vi "Human VOG.vi"(0 "3D (unticked 2D) processing":bool, 5 "Bin (unticked Mon) ocular processing":bool, 9 "Interpolate Timebase (Hz)":i32=250, 11 "Gyro scaling":dbl=200.0) -> (15 "Data Output":T1 {"Data Channels" format="%.2f"})   [LabVIEW 2013]
uses:
  <vilib>/Analysis/_algsub.llb/Real PseudoInverse Matrix.vi
  <vilib>/Utility/file.llb/Read From Spreadsheet File (DBL).vi
  comm/fick-matrix/fick-matrix.lvlib
  <vilib>/Analysis/NI_AALPro.lvlib
  comm/quaternion/quaternion.lvlib
panel:
  in  "stop":bool
  # "Human VOG System"
  # "By Americo Migliaccio 17-12-2008"
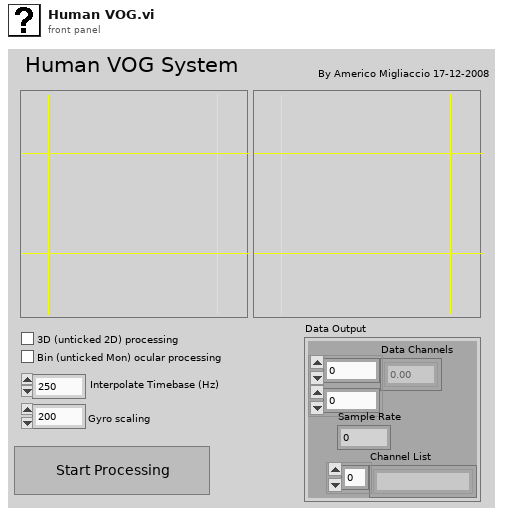
[diagram p1: front panel]
types:
  T1 = cluster{"Data Channels":dbl[][], "Sample Rate":i32, "Channel List":string[]}
  T2 = typedef "NI_Matrix.lvlib/RealMatrix.ctl" = dbl[][]
  T3 = cluster{dbl[][], "Interpolate Timebase (Hz)":i32, string[]}
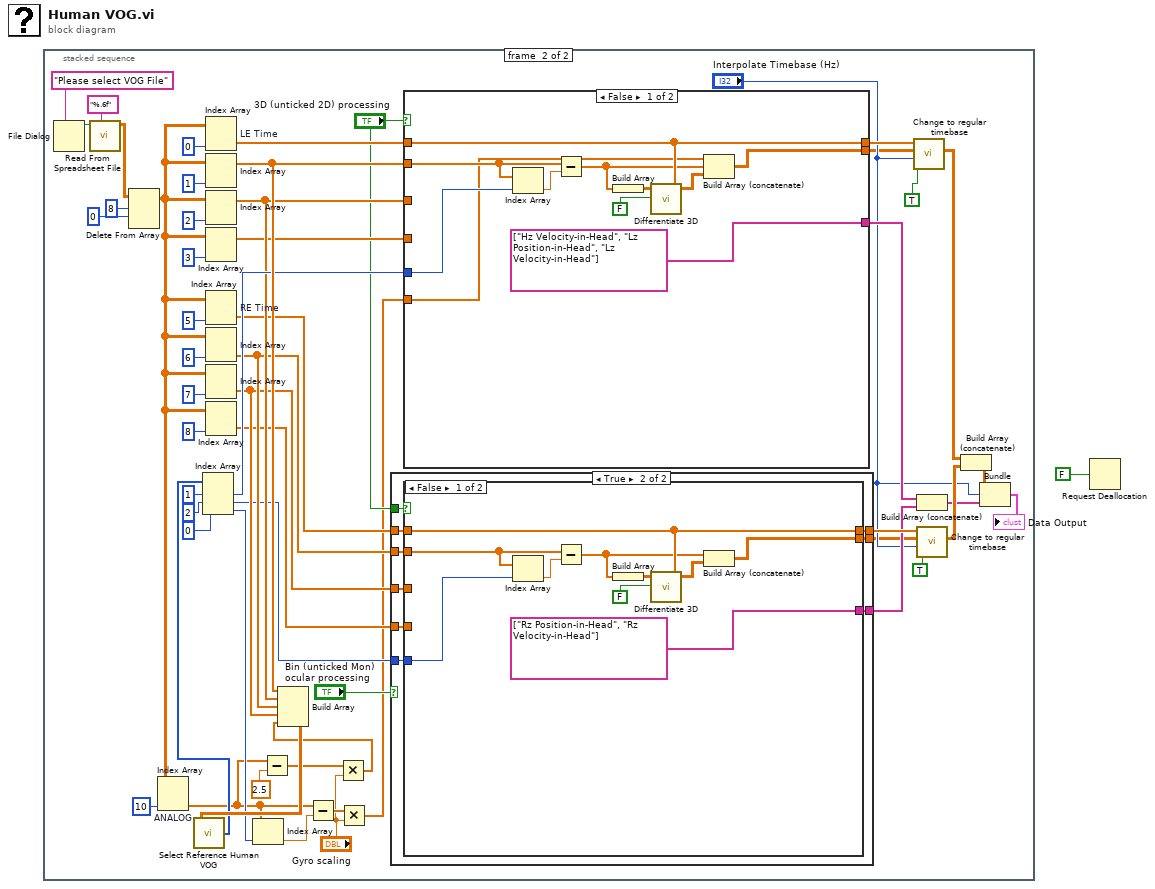
[diagram p0: block diagram]
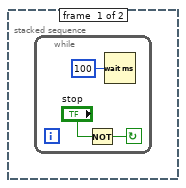
[diagram p2: hidden frame]
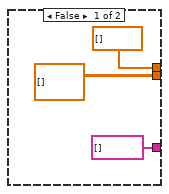
[diagram p3: hidden frame]
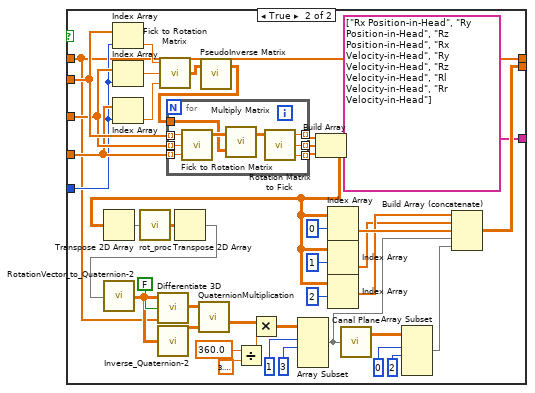
[diagram p4: hidden frame]
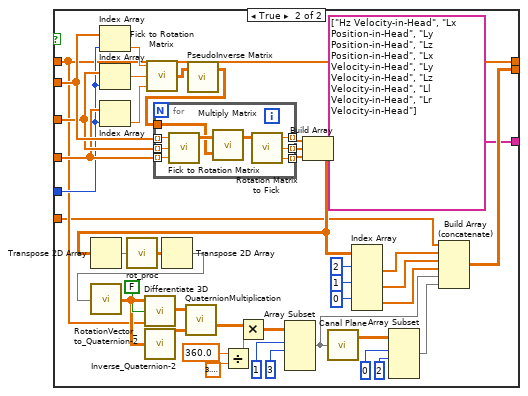
[diagram p5: hidden frame]
diagram:
  n1 = stacked-sequence {
    frame #0 {
      n2 = while {
        stop <- w2 continue-if-true
        n3 = Not(x="stop") -> (.not. x?=w2:bool)
        n4 = Wait (ms)(milliseconds to wait=u32 100) -> ()  [unwired: 1 out]
      }
    }
    frame #1 {
      n5 = File Dialog(7:"Please select VOG File" ("prompt")) -> (3:w51:path)  [unwired: 6 in, 3 out]
      n6 = call-poly <vilib>:"Read From Spreadsheet File.vi"("format (%.3f)"="%.6f", "file path (dialog if empty)"=w51) -> ("all rows"=w8:dbl[][])  [unwired: 5 in, 4 out]
      n7 = Delete From Array(array=w8, length=8 ("index"), index (row)=0) -> (array with subset deleted=w6:dbl[][])  [unwired: 1 in, 1 out]
      n8 = Index Array "ANALOG"(array=w6, index (col)=10 ("index (row)")) -> (element=w16:dbl[])  [unwired: 1 in]
      n9 = Index Array "LE Time"(array=w6, index (col)=0 ("index (row)")) -> (element=w47:dbl[])  [unwired: 1 in]
      n10 = Index Array(array=w6, index (col)=1 ("index (row)")) -> (element=w38:dbl[])  [unwired: 1 in]
      n11 = Index Array(array=w6, index (col)=2 ("index (row)")) -> (element=w35:dbl[])  [unwired: 1 in]
      n12 = Index Array(array=w6, index (col)=3 ("index (row)")) -> (element=w34:dbl[])  [unwired: 1 in]
      n13 = Index Array "RE Time"(array=w6, index (col)=5 ("index (row)")) -> (element=w33:dbl[])  [unwired: 1 in]
      n14 = Index Array(array=w6, index (col)=6 ("index (row)")) -> (element=w32:dbl[])  [unwired: 1 in]
      n15 = Index Array(array=w6, index (col)=7 ("index (row)")) -> (element=w31:dbl[])  [unwired: 1 in]
      n16 = Index Array(array=w6, index (col)=8 ("index (row)")) -> (element=w30:dbl[])  [unwired: 1 in]
      n17 = Subtract(x=w16, y=sgl 2.5 ("Array Index")) -> (x-y=w14:dbl[])
      n18 = Multiply(x=w14, y="Gyro scaling") -> (x*y=w12:dbl[])
      n19 = Build Array(w38, w35, w32, w31, w12) -> (w48:dbl[][])
      n20 = call "Select Reference Human VOG.vi"("3D Coil"=w48) -> ("References"=w41:i32[])
      n21 = Index Array ("RE Time")(array=w41, index #1=1 ("index"), index #2=2 ("index"), index #3=0 ("index")) -> (element #1=w37:i32, element #2=w29:i32, element #3=w36:i32)
      n22 = Index Array(array=w16, index=w36) -> (element=w40:dbl)
      n23 = Subtract(x=w16, y=w40) -> (x-y=w39:dbl[])
      n24 = Multiply(x=w39, y="Gyro scaling") -> (x*y=w24:dbl[])
      n25 = case shown="True" "Bin (unticked Mon) ocular processing" {
        tunnel: w33 -> [_ w72]
        tunnel: w32 -> [_ w71]
        tunnel: w31 -> [_ w70]
        tunnel: w30 -> [_ w69]
        tunnel: w29 -> [_ w68]
        tunnel: [dbl[][] [] w67] -> w9
        tunnel: [sgl[] [] ("all rows") w66] -> w27
        tunnel: "3D (unticked 2D) processing" -> [_ w65]
        tunnel: [string[] [] w64] -> w21
        frame False {
        }
        frame True {
          n26 = case shown="False" w65 {
            tunnel: w72 -> [w80 w84]
            tunnel: w71 -> [w76 w123]
            tunnel: [w80 w84] -> w66
            tunnel: [w78 w85] -> w67
            tunnel: w68 -> [w74 w120]
            tunnel: [string[] ["Rz Position-in-Head", "Rz Velocity-in-Head"] string[] ["Rx Position-in-Head", "Ry Position-in-Head", "Rz Position-in-Head", "Rx Velocity-in-Head", "Ry Velocity-in-Head", "Rz Velocity-in-Head", "Rl Velocity-in-Head", "Rr Velocity-in-Head"]] -> w64
            tunnel: w70 -> [_ w122]
            tunnel: w69 -> [_ w121]
            frame False {
              n27 = Index Array(array=w76, index=w74) -> (element=w77:dbl)
              n28 = Subtract(x=w76, y=w77) -> (x-y=w75:dbl[])
              n29 = Build Array(w75) -> (w81:dbl[][])
              n30 = call "Differentiate 3D.vi"("Timebase"=w80, "Fixed Sample Rate"=FALSE, "Data (in)"=w81) -> ("Data (differentiated)"=w79:dbl[][])  [unwired: 2 in]
              n31 = Build Array (concatenate)(w75, w79) -> (w78:dbl[][])
            }
            frame True {
              n32 = Index Array(array=w123, index=w120) -> (element=w117:dbl)
              n33 = Index Array(array=w122, index=w120) -> (element=w118:dbl)
              n34 = Index Array(array=w121, index=w120) -> (element=w119:dbl)
              n35 = call "Fick to Rotation Matrix.vi"("T"=w119, "V"=w118, "H"=w117) -> ("Rotation Matrix"=w116:dbl[][])
              n36 = call-poly <vilib>:"PseudoInverse Matrix.vi"("Input Matrix"=w116) -> ("PseudoInverse Matrix"=w115:T2)  [unwired: 1 in, 1 out]
              n37 = for {
                tunnel: w121 -> [w130] mode=indexing
                tunnel: w122 -> [w131] mode=indexing
                tunnel: w123 -> [w132] mode=indexing
                tunnel: [w128] -> w112 mode=indexing
                tunnel: [w127] -> w114 mode=indexing
                tunnel: [w126] -> w113 mode=indexing
                tunnel: w115 -> [w124]
                n38 = call "Fick to Rotation Matrix.vi"("T"=w130, "V"=w131, "H"=w132) -> ("Rotation Matrix"=w129:dbl[][])
                n39 = call "Multiply Matrix.vi"("1st rotation Matrix"=w124, "2nd rotation Matrix"=w129) -> ("Resultant Matrix"=w125:dbl[][])  [unwired: 1 in]
                n40 = call "Rotation Matrix to Fick.vi"("A"=w125) -> ("T"=w126:dbl, "V"=w127:dbl, "H"=w128:dbl)  [unwired: 2 in]
              }
              n41 = Divide(x=360.0, y=3.141592653589793) -> (x/y=w104:dbl)
              n42 = Build Array(w112, w114, w113) -> (w88:dbl[][])
              n43 = Transpose 2D Array(2D array=w88) -> (transposed array=w111:dbl[][])
              n44 = call "rot_proc.vi"("Euler Angles"=w111) -> ("Rotation Vectors"=w110:dbl[][])  [unwired: 17 in, 1 out]
              n45 = Transpose 2D Array(2D array=w110) -> (transposed array=w98:dbl[][])
              n46 = call "RotationVector_to_Quaternion-2.vi"("rotation vectors"=w98) -> ("quaternions"=w105:dbl[][])  [unwired: 4 in]
              n47 = call "Differentiate 3D.vi"("Timebase"=w84, "Fixed Sample Rate"=FALSE, "Data (in)"=w105) -> ("Data (differentiated)"=w99:dbl[][])  [unwired: 2 in]
              n48 = call "Inverse_Quaternion-2.vi"("quaternions"=w105) -> ("inverse quaternions"=w100:dbl[][])  [unwired: 4 in]
              n49 = call "QuaternionMultiplication.vi"("quaternions B"=w100, "quaternions A"=w99) -> ("quaternions A x B"=w101:dbl[][])  [unwired: 3 in]
              n50 = Multiply(x=w101, y=w104) -> (x*y=w109:dbl[][])
              n51 = Array Subset(array=w109, index (row)=1 ("Array Index"), length (row)=3 ("Array Index")) -> (w87:dbl[][])  [unwired: 2 in]
              n52 = Index Array(array=w88, index (row)=0) -> (element=w94:dbl[])  [unwired: 1 in]
              n53 = Index Array(array=w88, index (row)=1) -> (element=w92:dbl[])  [unwired: 1 in]
              n54 = Index Array(array=w88, index (row)=2) -> (element=w93:dbl[])  [unwired: 1 in]
              n55 = call "Canal Plane.vi"("Principal Planes"=w87) -> ("Canal Planes"=w95:dbl[][])
              n56 = Array Subset(array=w95, index (row)=0 ("Array Index"), length (row)=2 ("Array Index")) -> (w86:dbl[][])  [unwired: 2 in]
              n57 = Build Array (concatenate)(w93, w92, w94, w87, w86) -> (w85:dbl[][])
            }
          }
        }
      }
      n58 = case shown="False" "3D (unticked 2D) processing" {
        tunnel: w47 -> [w141 w151]
        tunnel: w38 -> [w139 w185]
        tunnel: [w141 w151] -> w46
        tunnel: [w134 w152] -> w10
        tunnel: w37 -> [w137 w182]
        tunnel: [string[] ["Hz Velocity-in-Head", "Lz Position-in-Head", "Lz Velocity-in-Head"] string[] ["Hz Velocity-in-Head", "Lx Position-in-Head", "Ly Position-in-Head", "Lz Position-in-Head", "Lx Velocity-in-Head", "Ly Velocity-in-Head", "Lz Velocity-in-Head", "Ll Velocity-in-Head", "Lr Velocity-in-Head"]] -> w22
        tunnel: w35 -> [_ w184]
        tunnel: w34 -> [_ w183]
        tunnel: w24 -> [w133 w144]
        frame False {
          n59 = Index Array(array=w139, index=w137) -> (element=w140:dbl)
          n60 = Subtract(x=w139, y=w140) -> (x-y=w138:dbl[])
          n61 = Build Array(w138) -> (w142:dbl[][])
          n62 = call "Differentiate 3D.vi"("Timebase"=w141, "Fixed Sample Rate"=FALSE, "Data (in)"=w142) -> ("Data (differentiated)"=w135:dbl[][])  [unwired: 2 in]
          n63 = Build Array (concatenate)(w133, w138, w135) -> (w134:dbl[][])
        }
        frame True {
          n64 = Index Array(array=w185, index=w182) -> (element=w179:dbl)
          n65 = Index Array(array=w184, index=w182) -> (element=w180:dbl)
          n66 = Index Array(array=w183, index=w182) -> (element=w181:dbl)
          n67 = call "Fick to Rotation Matrix.vi"("T"=w181, "V"=w180, "H"=w179) -> ("Rotation Matrix"=w178:dbl[][])
          n68 = call-poly <vilib>:"PseudoInverse Matrix.vi"("Input Matrix"=w178) -> ("PseudoInverse Matrix"=w177:T2)  [unwired: 1 in, 1 out]
          n69 = for {
            tunnel: w183 -> [w192] mode=indexing
            tunnel: w184 -> [w193] mode=indexing
            tunnel: w185 -> [w194] mode=indexing
            tunnel: [w190] -> w174 mode=indexing
            tunnel: [w189] -> w176 mode=indexing
            tunnel: [w188] -> w175 mode=indexing
            tunnel: w177 -> [w186]
            n70 = call "Fick to Rotation Matrix.vi"("T"=w192, "V"=w193, "H"=w194) -> ("Rotation Matrix"=w191:dbl[][])
            n71 = call "Multiply Matrix.vi"("1st rotation Matrix"=w186, "2nd rotation Matrix"=w191) -> ("Resultant Matrix"=w187:dbl[][])  [unwired: 1 in]
            n72 = call "Rotation Matrix to Fick.vi"("A"=w187) -> ("T"=w188:dbl, "V"=w189:dbl, "H"=w190:dbl)  [unwired: 2 in]
          }
          n73 = Divide(x=360.0, y=3.141592653589793) -> (x/y=w166:dbl)
          n74 = Build Array(w174, w176, w175) -> (w155:dbl[][])
          n75 = Transpose 2D Array(2D array=w155) -> (transposed array=w173:dbl[][])
          n76 = call "rot_proc.vi"("Euler Angles"=w173) -> ("Rotation Vectors"=w172:dbl[][])  [unwired: 17 in, 1 out]
          n77 = Transpose 2D Array(2D array=w172) -> (transposed array=w160:dbl[][])
          n78 = call "RotationVector_to_Quaternion-2.vi"("rotation vectors"=w160) -> ("quaternions"=w167:dbl[][])  [unwired: 4 in]
          n79 = call "Differentiate 3D.vi"("Timebase"=w151, "Fixed Sample Rate"=FALSE, "Data (in)"=w167) -> ("Data (differentiated)"=w161:dbl[][])  [unwired: 2 in]
          n80 = call "Inverse_Quaternion-2.vi"("quaternions"=w167) -> ("inverse quaternions"=w162:dbl[][])  [unwired: 4 in]
          n81 = call "QuaternionMultiplication.vi"("quaternions B"=w162, "quaternions A"=w161) -> ("quaternions A x B"=w163:dbl[][])  [unwired: 3 in]
          n82 = Multiply(x=w163, y=w166) -> (x*y=w171:dbl[][])
          n83 = Array Subset(array=w171, index (row)=1 ("Array Index"), length (row)=3 ("Array Index")) -> (w154:dbl[][])  [unwired: 2 in]
          n84 = call "Canal Plane.vi"("Principal Planes"=w154) -> ("Canal Planes"=w157:dbl[][])
          n85 = Index Array(array=w155, index (row) #1=2 ("index (row)"), index (row) #2=1 ("index (row)"), index (row) #3=0 ("index (row)")) -> (element #1=w147:dbl[], element #2=w146:dbl[], element #3=w145:dbl[])  [unwired: 3 in]
          n86 = Array Subset(array=w157, index (row)=0 ("Array Index"), length (row)=2 ("Array Index")) -> (w153:dbl[][])  [unwired: 2 in]
          n87 = Build Array (concatenate)(w144, w147, w146, w145, w154, w153) -> (w152:dbl[][])
        }
      }
      n88 = call "Change to regular timebase.vi"("NaN (unticked Interpolate)"=TRUE ("NaN"), "Sample Rate"="Interpolate Timebase (Hz)", "Data"=w10, "Time"=w46) -> ("Interp Data"=w11:dbl[][])  [unwired: 6 in]
      n89 = Build Array (concatenate)(w22, w21) -> (w18:string[])
      n90 = call "Change to regular timebase.vi"("NaN (unticked Interpolate)"=TRUE ("NaN"), "Sample Rate"="Interpolate Timebase (Hz)", "Data"=w9, "Time"=w27) -> ("Interp Data"=w23:dbl[][])  [unwired: 6 in]
      n91 = Build Array (concatenate)(w11, w23) -> (w20:dbl[][])
      n92 = Bundle(w20, "Interpolate Timebase (Hz)"="Interpolate Timebase (Hz)", w18) -> (→"Data Output":T3)  [unwired: 1 in]
    }
  }
  n93 = Request Deallocation(FALSE ("flag")) -> ()
